vi "S2DS_ConfigReadDC (SubVI).vi"(0 "Refnum in":T3, 1 "DC Info list (in)":T1, 3 "error in (no error)":errorcluster) -> (6 "Refnum out":T3, 7 "DC Info list (out)":T1, 9 "error out":errorcluster)   [LabVIEW 2025]
uses:
  <vilib>/Utility/config.llb/Config Data RefNum.ctl
  TYPE DEFS/S2DS_DAC info new.ctl
  TYPE DEFS/S2DS_Single DC info.ctl
  <vilib>/Utility/config.llb/Read Key (U32).vi
  <vilib>/Utility/config.llb/Read Key (String).vi
  <vilib>/Utility/config.llb/Read Key (Double).vi
  <vilib>/Utility/config.llb/NI_LVConfig.lvlib
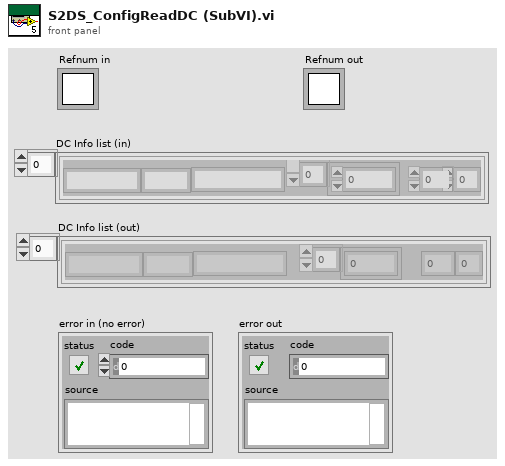
[diagram p1: front panel]
types:
  T1 = typedef "S2DS_DAC info new.ctl" = T2[]
  T2 = typedef "S2DS_Single DC info.ctl" = cluster{"Operation identifier":string, "DC parameters":dbl[], "U":i32, "V":i32, "Name":string, "Unit":string}
  T3 = typedef "NI_LVConfig.lvlib/Config Data RefNum.ctl" = refnum<k1>
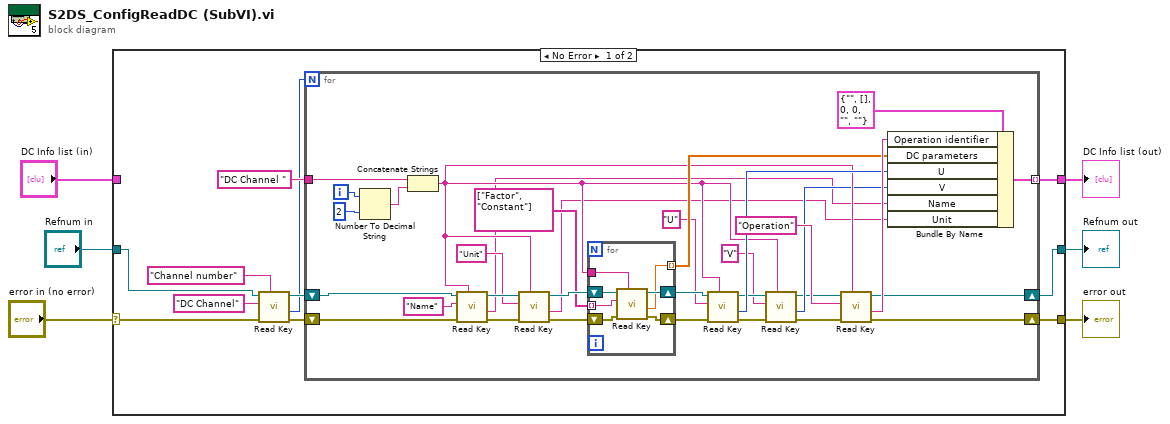
[diagram p0: block diagram]
diagram:
  n1 = case shown="No Error" "error in (no error)" {
    selector: "error in (no error)" -> [w8 w59]
    tunnel: [w17 w59] -> w6
    tunnel: [w16 w60] -> w5
    tunnel: [w14 w58] -> w4
    tunnel: "Refnum in" -> [w7 w60]
    tunnel: "DC Info list (in)" -> [_ w58]
    frame No Error {
      n2 = call-poly <vilib>:"Read Key.vi"("section"="Channel number", "error in (no error)"=w8, "key"="DC Channel", "refnum"=w7) -> ("error out"=w12:errorcluster, "value"=w9:u32, "refnum out"=w13:T3)  [unwired: 1 in, 4 out]
      n3 = for {
        N: w9 -> [_]
        shift-right: [w35] -> w16
        shift-left: w13 -> [w50]
        shift-right: [w34] -> w17
        shift-left: w12 -> [w49]
        tunnel: "DC Channel " -> [w45]
        tunnel: [w38] -> w14 mode=indexing
        i -> [w46]
        n4 = Number To Decimal String(number=w46, width (-)=i16 2) -> (decimal integer string=w48:string)
        n5 = Concatenate Strings(w45, w48) -> (w26:string)
        n6 = call-poly <vilib>:"Read Key.vi"("section"=w26, "error in (no error)"=w49, "key"="Name", "refnum"=w50) -> ("error out"=w42:errorcluster, "value"=w19:string, "refnum out"=w43:T3)  [unwired: 2 in, 3 out]
        n7 = call-poly <vilib>:"Read Key.vi"("section"=w26, "error in (no error)"=w42, "key"="Unit", "refnum"=w43) -> ("error out"=w40:errorcluster, "value"=w18:string, "refnum out"=w39:T3)  [unwired: 2 in, 3 out]
        n8 = for {
          tunnel: string[] ["Factor", "Constant"] -> [w53] mode=indexing
          shift-right: [w54] -> w30
          shift-left: w40 -> [w56]
          shift-right: [w55] -> w31
          shift-left: w39 -> [w57]
          tunnel: [w52] -> w32 mode=indexing
          tunnel: w26 -> [w51]
          n9 = call-poly <vilib>:"Read Key.vi"("section"=w51, "error in (no error)"=w56, "key"=w53, "refnum"=w57) -> ("error out"=w54:errorcluster, "value"=w52:dbl, "refnum out"=w55:T3)  [unwired: 1 in, 4 out]
        }
        n10 = call-poly <vilib>:"Read Key.vi"("section"=w26, "error in (no error)"=w30, "key"="U", "refnum"=w31) -> ("error out"=w21:errorcluster, "value"=w28:u32, "refnum out"=w27:T3)  [unwired: 1 in, 4 out]
        n11 = call-poly <vilib>:"Read Key.vi"("section"=w26, "error in (no error)"=w21, "key"="V", "refnum"=w27) -> ("error out"=w23:errorcluster, "value"=w25:u32, "refnum out"=w24:T3)  [unwired: 1 in, 4 out]
        n12 = call-poly <vilib>:"Read Key.vi"("section"=w26, "error in (no error)"=w23, "key"="Operation", "refnum"=w24) -> ("error out"=w34:errorcluster, "value"=w36:string, "refnum out"=w35:T3)  [unwired: 2 in, 3 out]
        n13 = Bundle By Name(cluster=T2 {"Operation identifier"="", "DC parameters"=[], "U"=0, "V"=0, "Name"="", "Unit"=""} ("Write channel info"), "Operation identifier"=w36, "DC parameters"=w32, "U"=w28, "V"=w25, "Name"=w19, "Unit"=w18) -> (w38:T2)
      }
    }
    frame Error {
    }
  }
  "error out" <- w6
  "Refnum out" <- w5
  "DC Info list (out)" <- w4
